vi "endEventToString.vi"(8 "error in (no error)":errorcluster, 11 "RampToneAmplitudeDown in":refnum<class "RampToneAmplitudeDown.lvclass">) -> (0 "error out":errorcluster, 2 "eventStringArray":string[](array[string]), 3 "RampToneAmplitudeDown out":refnum<class "RampToneAmplitudeDown.lvclass">)   [LabVIEW 2009, in "Tools.lvlib" / "Scripting.lvlib" / "RampToneAmplitudeDown.lvclass"]
uses:
  RampToneAmplitudeDown.lvclass
  SingleTone/SingleTone.lvclass
  RampTone/RampTone.lvclass
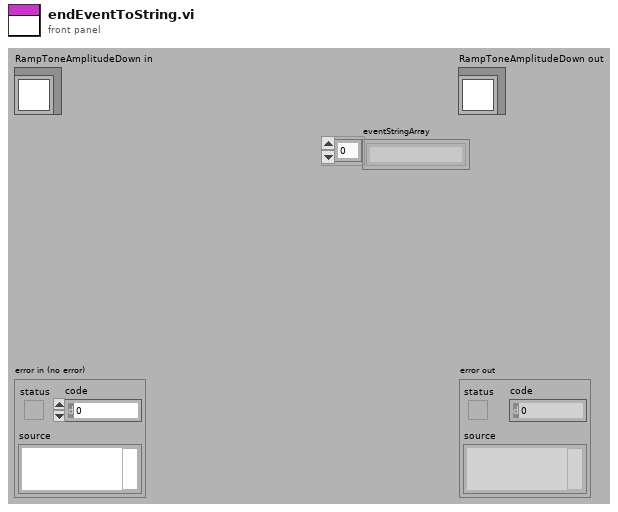
[diagram p1: front panel]
types:
  T1 = cluster{"rampTime":dbl, "timeStep":dbl, "dataValueStep":dbl}
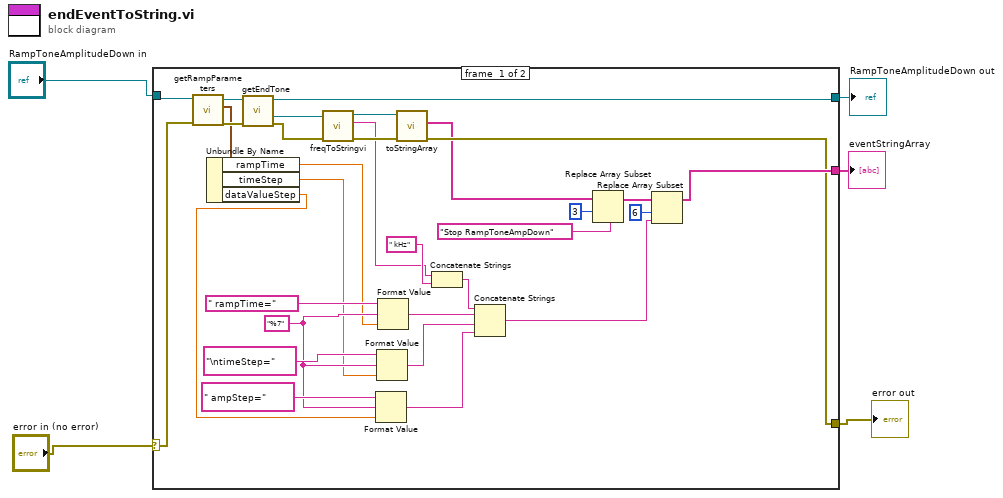
[diagram p0: block diagram]
diagram:
  n1 = case shown="No Error" "error in (no error)" {
    selector: "error in (no error)" -> [w15 w37]
    tunnel: [w20 w37] -> w2
    tunnel: [w26 _] -> w1
    tunnel: "RampToneAmplitudeDown in" -> [w16 w38]
    tunnel: [w11 w38] -> w3
    frame #0 {
      w25 = "%7"
      n2 = call "getRampParameters.vi"("error in (no error)"=w15, "RampTone in"=w16) -> ("error out"=w14:errorcluster, "RampParameters"=w9:T1, "RampTone out"=w13:refnum<class "RampToneAmplitudeDown.lvclass">)  [unwired: 7 in]
      n3 = Unbundle By Name(w9) -> ("rampTime"=w8:dbl, "timeStep"=w7:dbl, "dataValueStep"=w6:dbl)
      n4 = call-dynamic "getEndTone.vi"("error in (no error)"=w14, "RampTone.lvclass in"=w13) -> ("error out"=w10:errorcluster, "endTone.lvclass"=w12:refnum<class "SingleTone.lvclass">, "RampTone.lvclass out"=w11:refnum<class "RampToneAmplitudeDown.lvclass">)  [unwired: 7 in]
      n5 = call-dynamic "freqToStringvi.vi"("error in (no error)"=w10, "SingleTone in"=w12) -> ("error out"=w21:errorcluster, "frequency"=w18:string, "SingleTone out"=w17:refnum<class "SingleTone.lvclass">)  [unwired: 7 in]
      n6 = Format Value(string ("")=" ampStep=", format string=w25, value (0)=w6) -> (output string=w22:string)
      n7 = Format Value(string ("")="\ntimeStep=", format string=w25, value (0)=w7) -> (output string=w28:string)
      n8 = Format Value(string ("")=" rampTime=", format string=w25, value (0)=w8) -> (output string=w29:string)
      n9 = call-dynamic "toStringArray.vi"("error in (no error)"=w21, "SingleTone in"=w17) -> ("error out"=w20:errorcluster, "eventStringArray"=w19:string[])  [unwired: 7 in, 1 out]
      n10 = Concatenate Strings(w18, " kHz") -> (w23:string)
      n11 = Concatenate Strings(w23, w29, w28, w22) -> (w27:string)
      n12 = Replace Array Subset(array=w19, new element="Stop RampToneAmpDown", index=3) -> (w32:string[])
      n13 = Replace Array Subset(array=w32, new element=w27, index=6) -> (w26:string[])
    }
    frame #1 {
    }
  }
  "error out" <- w2
  "RampToneAmplitudeDown out" <- w3
  "eventStringArray" <- w1
